vi "矩阵操作.vi"() -> ()   [LabVIEW 2018]
uses:
  <vilib>/Analysis/Matrix/Datatypes/RealMatrix.ctl
  <vilib>/Analysis/baseanly.llb/Real Dot Product.vi
  <vilib>/Analysis/Matrix/Numeric/Add/Add - RM,RM.vi
  <vilib>/Analysis/Matrix/NI_Matrix.lvlib
  <vilib>/Analysis/NI_AALBase.lvlib
panel:
  in  "停止":bool
  in  "?":T1(tab)
  in  "数组":dbl[](array[numeric])
  in  "数组 2":dbl[](array[numeric])
  out "数组 3":dbl[](array[numeric])
  out "Real Matrix 3":T2 caption="实数矩阵3"
  in  "Real Matrix 2":T2 caption="实数矩阵2"
  in  "Real Matrix":T2 caption="实数矩阵"
  out "簇 3":cluster{"数值":dbl, "数值 2":dbl, "数组":dbl[]}
  in  "簇 2":cluster{"数值":dbl, "数值 2":dbl, "数组":dbl[]}
  in  "簇":cluster{"数值":dbl, "数值 2":dbl, "数组":dbl[]}
  out "数组 5":dbl[](array[numeric])
  in  "数值":dbl
  in  "数组 4":dbl[](array[numeric])
  in  "X Vector":dbl[](array[numeric]) caption="X向量" format="%.2f"
  in  "Y Vector":dbl[](array[numeric]) caption="Y向量" format="%.2f"
  out "X * Y":dbl format="%.2f"
  out "波形图 2":dbl[](graph)
  out "波形图":dbl[](graph)
  in  "数组 6":dbl[](array[numeric])
  # "+"
  # "="
  # "+"
  # "="
  # "+"
  # "="
  # "+"
  # "="
  # "·"
  # "="
  # "+"
  # "="
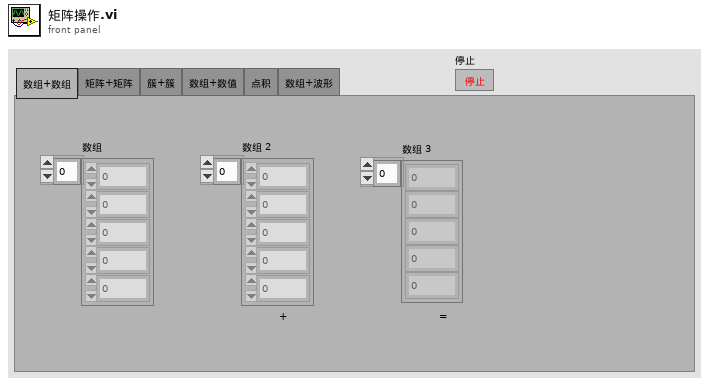
[diagram p1: front panel]
types:
  T1 = enum32{"数组+数组", "矩阵+矩阵", "簇+簇", "数组+数值", "点积", "数组+波形"}
  T2 = typedef "NI_Matrix.lvlib/RealMatrix.ctl" = dbl[][]
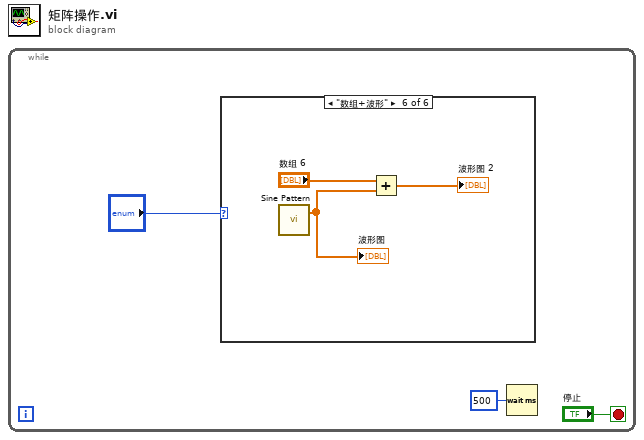
[diagram p0: block diagram]
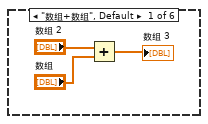
[diagram p2: hidden frame]
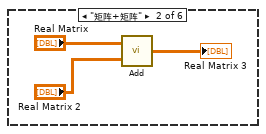
[diagram p3: hidden frame]
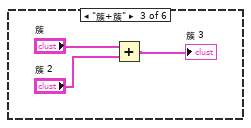
[diagram p4: hidden frame]
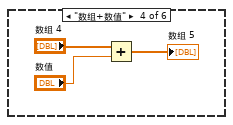
[diagram p5: hidden frame]
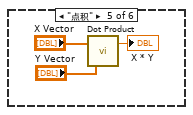
[diagram p6: hidden frame]
diagram:
  n1 = while {
    stop <- "停止" stop-if-true
    n2 = case shown="\"数组+波形\"" "?" {
      frame "数组+数组", Default {
        n3 = Add(x="数组 2", y="数组") -> (x+y=→"数组 3":dbl[])
      }
      frame "矩阵+矩阵" {
        n4 = call-poly <vilib>:"Add.vi"("Real Matrix B"="Real Matrix 2", "Real Matrix A"="Real Matrix") -> ("A + B"=→"Real Matrix 3":T2)
      }
      frame "簇+簇" {
        n5 = Add(x="簇", y="簇 2") -> (x+y=→"簇 3":cluster{"数值":dbl, "数值 2":dbl, "数组":dbl[]})
      }
      frame "数组+数值" {
        n6 = Add(x="数组 4", y="数值") -> (x+y=→"数组 5":dbl[])
      }
      frame "点积" {
        n7 = call-poly <vilib>:"Dot Product.vi"("Y Vector"="Y Vector", "X Vector"="X Vector") -> ("X * Y"=→"X * Y":dbl)  [unwired: 1 out]
      }
      frame "数组+波形" {
        n8 = call <vilib>:"Sine Pattern.vi"() -> ("Sinusoidal Pattern"=w19:dbl[])  [unwired: 4 in, 1 out]
        "波形图" <- w19
        n9 = Add(x="数组 6", y=w19) -> (x+y=→"波形图 2":dbl[])
      }
    }
    n10 = Wait (ms)(milliseconds to wait=u32 500 ("等待时间（毫秒）")) -> ()  [unwired: 1 out]
  }
